vi "ZY_Relay.vi"(6 "Addr":string, 7 "Read?":bool=TRUE, 8 "error in (no error)":errorcluster, 9 "ON?":bool, 10 "Channel":string, 11 "VISA resource name":refnum<visa-resource-name>) -> (0 "error out":errorcluster, 2 "read buffer":string)   [LabVIEW 2013]
uses:
  <vilib>/Instr/_visa.llb/VISA Flush IO Buffer Mask.ctl
  <vilib>/Instr/_visa.llb/VISA Configure Serial Port (Instr).vi
panel:
  out "concatenated string":string
  in  "wait ms":i32=100
  out "CMD":string
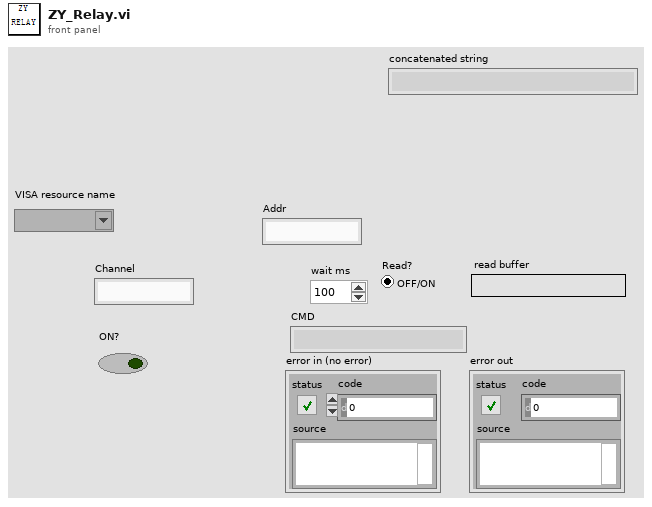
[diagram p1: front panel]
types:
  T1 = typedef "VISA Flush IO Buffer Mask.ctl" = u16
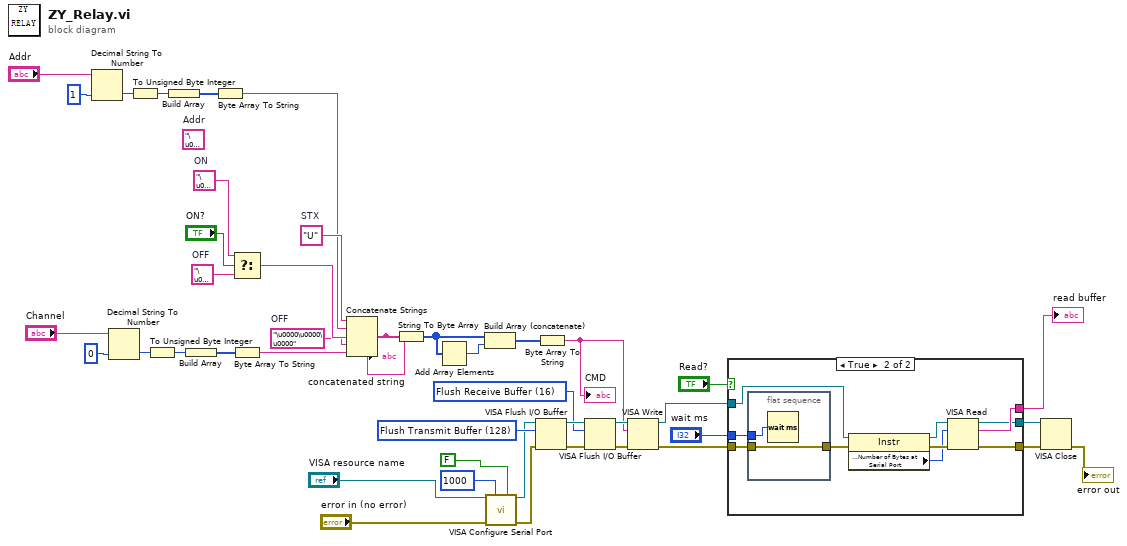
[diagram p0: block diagram]
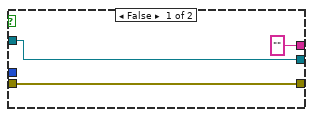
[diagram p2: hidden frame]
diagram:
  w19 = T1 16 items=["Flush Receive Buffer"=16, "Write Transmit Buffer to Device"=32, "Flush Receive Buffer (No I/O)"=64, "Flush Transmit Buffer"=128] ("Mask")
  w20 = T1 128 items=["Flush Receive Buffer"=16, "Write Transmit Buffer to Device"=32, "Flush Receive Buffer (No I/O)"=64, "Flush Transmit Buffer"=128] ("Mask")
  w34 = "\u0000\u0000\u0000"  # OFF
  w38 = "\u0011"  # OFF
  w37 = "\u0012"  # ON
  (unwired) "\u0001"  # Addr
  w39 = "U"  # STX
  n1 = Decimal String To Number(string="Addr", default (0L)=1 ("default (0 I32)")) -> (number=w3:i32)  [unwired: 1 in, 1 out]
  n2 = Decimal String To Number(string="Channel", default (0L)=0 ("default (0 I32)")) -> (number=w31:i32)  [unwired: 1 in, 1 out]
  n3 = To Unsigned Byte Integer(number=w3) -> (unsigned 8bit integer=w6:u8)
  n4 = To Unsigned Byte Integer(number=w31) -> (unsigned 8bit integer=w28:u8)
  n5 = Build Array(w6) -> (w2:u8[])
  n6 = Build Array(w28) -> (w33:u8[])
  n7 = Byte Array To String(unsigned byte array=w2) -> (string=w1:string)
  n8 = Select(t=w37, s="ON?", f=w38) -> (s? t:f=w36:string)
  n9 = Byte Array To String(unsigned byte array=w33) -> (string=w32:string)
  n10 = Concatenate Strings(w39, w1, w36, w34, w32) -> (w40:string)
  "concatenated string" <- w40
  n11 = String To Byte Array(string=w40) -> (unsigned byte array=w43:u8[])
  n12 = Add Array Elements(numeric array=w43) -> (sum=w42:u8)
  n13 = Build Array (concatenate)(w43, w42) -> (w41:u8[])
  n14 = call-poly "VISA Configure Serial Port"("VISA resource name"="VISA resource name", "timeout (10sec)"=1000 ("wait ms"), "Enable Termination\nChar (T)"=FALSE ("Enable Termination\nChar (T)"), "error in (no error)"="error in (no error)") -> ("VISA resource name out"=w12:refnum<visa-resource-name>, "error out"=w15:errorcluster)  [unwired: 10 in]
  n15 = VISA Flush I/O Buffer(VISA resource name=w12, mask (16)=w20, error in (no error)=w15) -> (VISA resource name out=w21:refnum<visa-resource-name>, error out=w17:errorcluster)
  n16 = Byte Array To String(unsigned byte array=w41) -> (string=w11:string)
  "CMD" <- w11
  n17 = VISA Flush I/O Buffer(VISA resource name=w21, mask (16)=w19, error in (no error)=w17) -> (VISA resource name out=w18:refnum<visa-resource-name>, error out=w16:errorcluster)
  n18 = VISA Write(VISA resource name=w18, write buffer=w11, error in (no error)=w16) -> (VISA resource name out=w25:refnum<visa-resource-name>, error out=w23:errorcluster)  [unwired: 1 out]
  n19 = case shown="True" "Read?" {
    tunnel: ["" ("read buffer") w56] -> w7
    tunnel: [w45 w55] -> w10
    tunnel: [w46 w54] -> w8
    tunnel: w25 -> [w46 w51]
    tunnel: "wait ms" -> [_ w50]
    tunnel: w23 -> [w45 w48]
    frame False {
    }
    frame True {
      n20 = flat-sequence {
        tunnel: w50 -> [w58]
        tunnel: [w57] -> w49
        tunnel: w48 -> [w57]
        frame #0 {
          n21 = Wait (ms)(milliseconds to wait=w58) -> ()  [unwired: 1 out]
        }
      }
      n22 = property class="Instr"(reference=w51, error in=w49) -> (reference out=w52:refnum<visa-resource-name>, error out=w53:errorcluster, "Serial Settings:Number of Bytes at Serial Port"=w47:u32)
      n23 = VISA Read(VISA resource name=w52, byte count=w47, error in (no error)=w53) -> (VISA resource name out=w54:refnum<visa-resource-name>, read buffer=w56:string, error out=w55:errorcluster)  [unwired: 1 out]
    }
  }
  "read buffer" <- w7
  n24 = VISA Close(VISA resource name=w8, error in (no error)=w10) -> (error out=→"error out":errorcluster)
